vi "GL_MHeaterDisplay.vi"() -> ()   [LabVIEW 2021]
panel:
  out "MANUAL HEATER DISPLAY":dbl(slide) caption="AMP" min=0.0 max=5.0 scale=0.0..5.0
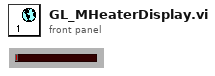
[diagram p1: front panel]
diagram:
